vi "trigger_rising_edge_diag_dctime.vi"(10 "Ref_MLD measurement":dbl[][](array[numeric]), 11 "dt in":dbl) -> (3 "Waveform":waveform(dbl), 4 "First Rising edge index":i32, 6 "Frequency":dbl, 7 "Ref_MLD_triggered":dbl[][](array[numeric]))   [LabVIEW 2013]
uses:
  <vilib>/Analysis/baseanly.llb/Mean (DBL).vi
  <vilib>/Analysis/NI_AALBase.lvlib
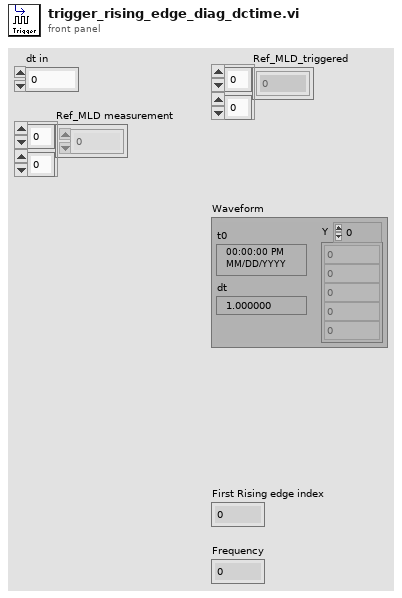
[diagram p1: front panel]
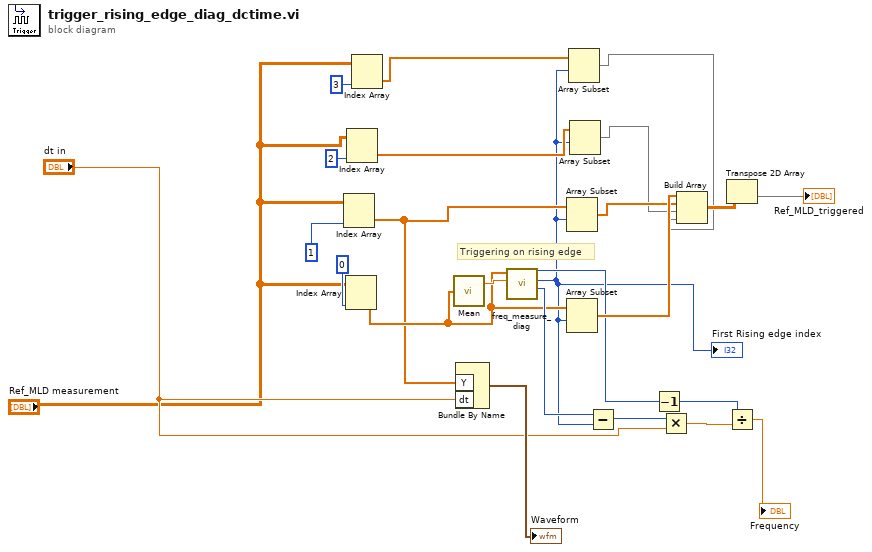
[diagram p0: block diagram]
diagram:
  # "Triggering on rising edge"
  n1 = Index Array(array="Ref_MLD measurement", index (col)=1 ("index (row)")) -> (element=w9:dbl[])  [unwired: 1 in]
  n2 = Index Array(array="Ref_MLD measurement", index (col)=0 ("index (row)")) -> (element=w10:dbl[])  [unwired: 1 in]
  n3 = Index Array(array="Ref_MLD measurement", index (col)=2 ("disabled index (col)")) -> (element=w5:dbl[])  [unwired: 1 in]
  n4 = Index Array(array="Ref_MLD measurement", index (col)=3 ("disabled index (col)")) -> (element=w4:dbl[])  [unwired: 1 in]
  n5 = call-poly <vilib>:"Mean.vi"("X"=w10) -> ("mean"=w19:dbl)  [unwired: 1 out]
  n6 = Bundle By Name("Y"=w9, "dt"="dt in") -> (→"Waveform":waveform(dbl))  [unwired: 1 in]
  n7 = call "freq_measure_diag.vi"("Ref_average"=w19, "data"=w10) -> ("Actual (last) Rising edge index"=w15:i32, "First Rising edge index"=w3:i32, "Rising edges"=w12:i32)  [unwired: 7 in]
  "First Rising edge index" <- w3
  n8 = Array Subset(array=w9, index=w3) -> (w22:dbl[])  [unwired: 1 in]
  n9 = Array Subset(array=w10, index=w3) -> (w23:dbl[])  [unwired: 1 in]
  n10 = Array Subset(array=w4, index=w3) -> (w1:dbl[])  [unwired: 1 in]
  n11 = Array Subset(array=w5, index=w3) -> (w2:dbl[])  [unwired: 1 in]
  n12 = Subtract(x=w15, y=w3) -> (x-y=w17:i32)
  n13 = Decrement(x=w12) -> (x-1=w11:i32)
  n14 = Multiply(x=w17, y="dt in") -> (x*y=w16:dbl)
  n15 = Build Array(w23, w22, w2, w1) -> (w24:dbl[][])
  n16 = Transpose 2D Array(2D array=w24) -> (transposed array=→"Ref_MLD_triggered":dbl[][])
  n17 = Divide(x=w11, y=w16) -> (x/y=→"Frequency":dbl)
